vi "Read Inclinometer Obj.vi"(8 "error in (no error)":errorcluster, 11 "Inclinometer Configuration in":refnum<class "Inclinometer Configuration.lvclass">) -> (0 "error out":errorcluster, 2 "Hardware.lvlib:Inclinometer.lvlib:Inclinometer.lvclass":refnum<class "Inclinometer.lvclass">, 3 "Inclinometer Configuration out":refnum<class "Inclinometer Configuration.lvclass">)   [LabVIEW 2016, in "Hardware.lvlib" / "Inclinometer.lvlib" / "Inclinometer Configuration.lvclass"]
uses:
  <userlib>/Common Components/Hardware/Inclinometer/Inclinometer Config/Inclinometer Configuration.lvclass
  <userlib>/Common Components/Hardware/Inclinometer/Inclinometer/Inclinometer.lvclass
  <userlib>/Common Components/Hardware/Inclinometer/Inclinometer Config/Inclinometer Configuration.lvclass/Inclinometer Configuration.ctl
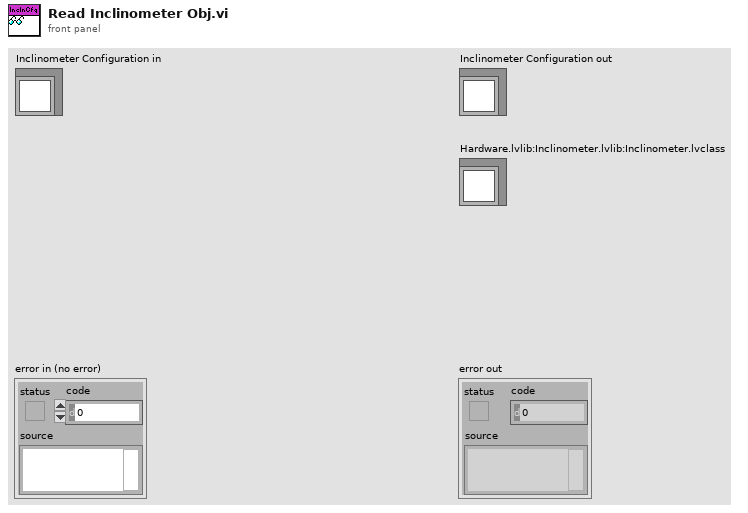
[diagram p1: front panel]
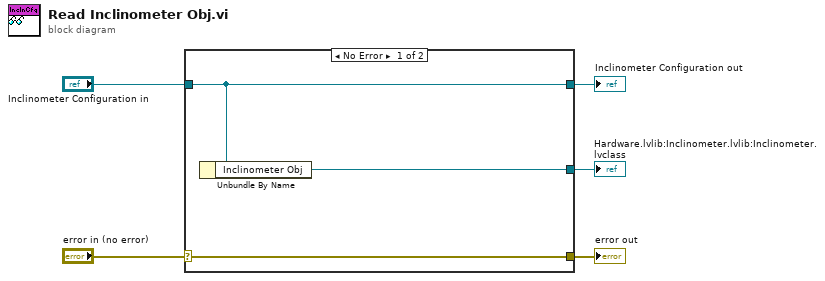
[diagram p0: block diagram]
diagram:
  n1 = case shown="No Error" "error in (no error)" {
    selector: "error in (no error)" -> [w8 w9]
    tunnel: [w8 w9] -> w4
    tunnel: [w7 w10] -> w2
    tunnel: "Inclinometer Configuration in" -> [w7 w10]
    tunnel: [w6 _] -> w1
    frame No Error {
      n2 = Unbundle By Name(w7) -> ("Inclinometer Obj"=w6:refnum<class "Inclinometer.lvclass">)
    }
    frame Error {
    }
  }
  "error out" <- w4
  "Inclinometer Configuration out" <- w2
  "Hardware.lvlib:Inclinometer.lvlib:Inclinometer.lvclass" <- w1
